vi "Charger_VBAT Init.vi"(6 "VBAT refnum":refnum<vi>, 7 "Status Refnum  Array":T1[](array[typedef]), 8 "error in":errorcluster) -> (0 "error out":errorcluster)   [LabVIEW 2020]
doc: "This function initializes the RUN, STOP, and PRINT button \"Value\" and \"Disabled\" attributes."
uses:
  Charger_Status Refnum.ctl
  Drivers/Charger Test Set/Charger_Input Control.ctl
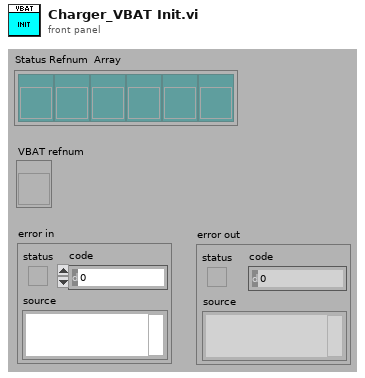
[diagram p1: front panel]
types:
  T1 = typedef "Charger_Status Refnum.ctl" = refnum<vi>
  T2 = typedef "Charger_Input Control.ctl" = cluster{"address":refnum<visa-resource-name>, "position":i32, "setpoint":dbl}
  T3 = cluster{"MICS ID":u32, "VBAT":dbl, "ChargingState":string, "VBAT Slide":dbl, "Status":string, "TemperatureLevel":dbl, "IPG_ReceivedLevel":dbl, "VBAT Target":dbl, "Charger Setpoint":dbl, "Index":i32, "Ready":bool, "Charger Inputs":T2, "MICS Inputs":cluster{"address":refnum<visa-resource-name>, "chan":u16, "ID":u32}}
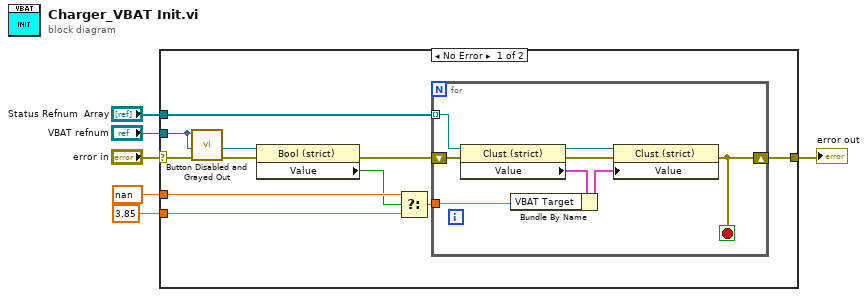
[diagram p0: block diagram]
diagram:
  n1 = case shown="No Error" "error in" {
    selector: "error in" -> [w16 w25]
    tunnel: [w11 w25] -> w6
    tunnel: "VBAT refnum" -> [w14 _]
    tunnel: "Status Refnum  Array" -> [w13 _]
    tunnel: nan -> [w10 _]
    tunnel: 3.85 -> [w9 _]
    frame No Error {
      n2 = call "Button Disabled and Grayed Out.vi"("error in"=w16, "button refnum"=w14) -> ("error out"=w15:errorcluster)  [unwired: 6 in, 1 out]
      n3 = property class="Bool (strict)"(reference=w14, error in=w15) -> (error out=w12:errorcluster, "Value"=w7:bool)  [unwired: 1 out]
      n4 = Select(t=w10, s=w7, f=w9) -> (s? t:f=w8:dbl)
      n5 = for {
        shift-right: [w19] -> w11
        shift-left: w12 -> [w24]
        tunnel: w13 -> [w23] mode=indexing
        tunnel: w8 -> [w18]
        stop <- w19 stop-if-true
        n6 = property class="Clust (strict)"(reference=w23, error in=w24) -> (reference out=w17:T1, error out=w22:errorcluster, "Value"=w20:T3)
        n7 = Bundle By Name(cluster=w20, "VBAT Target"=w18) -> (w21:T3)
        n8 = property class="Clust (strict)"(reference=w17, error in=w22, "Value"=w21) -> (error out=w19:errorcluster)  [unwired: 1 out]
      }
    }
    frame Error {
    }
  }
  "error out" <- w6
